vi "prob2.vi"() -> ()   [LabVIEW 2022 SP3]
uses:
  <vilib>/express/express analysis/Spectral/Block/exnSpectralBlock spectral measurements power poly.vi
  <vilib>/express/express analysis/Spectral/Block/exnSpectralBlock spectral measurements power DDT.vi
  <vilib>/express/express analysis/Spectral/XNode/ExpressSpectralMeasurementsBlockNode.xnode
panel:
  in  "stop":bool
  out "Waveform Graph 6":dynamicdata(graph)
  out "Waveform Graph 5":dynamicdata(graph)
  out "Filtered Signal":dynamicdata(graph)
  in  "Cutoff Frequency":dbl(slide) scale=0.0..1000.0
  out "Raw Signal":dynamicdata(graph)
  out "Channel 2":dynamicdata(graph)
  in  "Amplitude":dbl(slide) scale=0.0..10.0
  in  "Frequency":dbl(knob) scale=0.0..1000.0
  out "Channel 1":dynamicdata(graph)
  in  "Amplitude":dbl(slide) scale=0.0..10.0
  in  "Frequency":dbl(knob) scale=0.0..1000.0
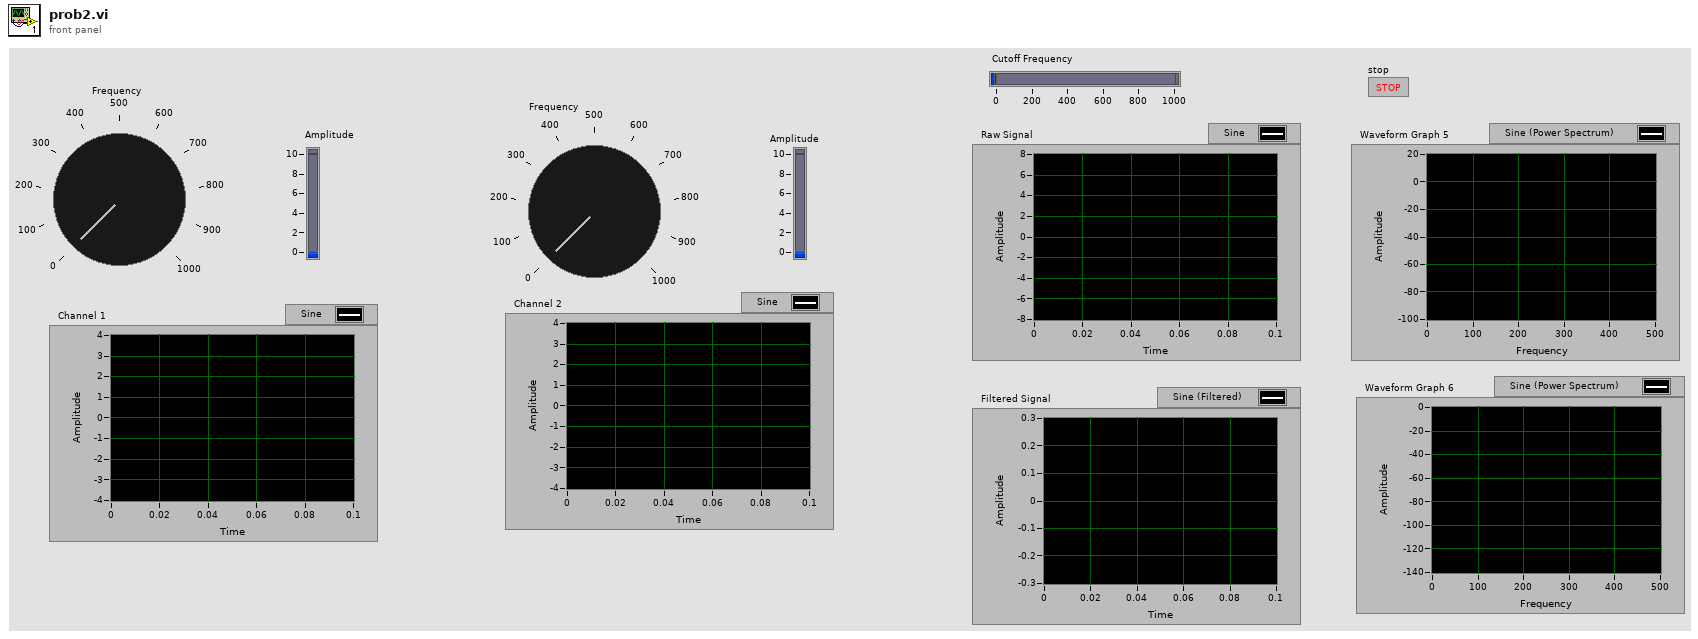
[diagram p1: front panel]
types:
  T1 = cluster{"averaging mode":u16, "weighting mode":u16, "number of averages":u32}
  T2 = cluster{"dB On (F)":bool, "unwrap phase (F)":bool, "convert to degree (F)":bool}
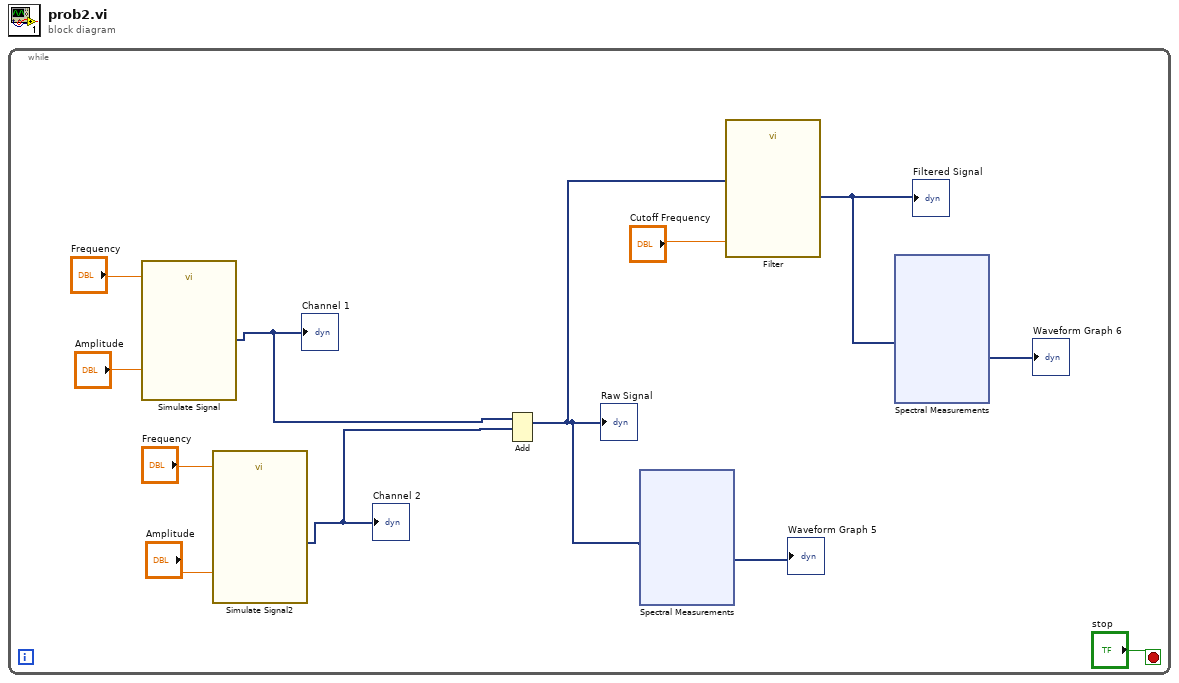
[diagram p0: block diagram]
diagram:
  n1 = while {
    stop <- "stop" stop-if-true
    n2 = call "Simulate Signal"("Frequency"="Frequency", "Amplitude"="Amplitude") -> ("Sine"=w8:dynamicdata)  [unwired: 12 in, 1 out]
    "Channel 1" <- w8
    n3 = call "Simulate Signal2"("Frequency"="Frequency", "Amplitude"="Amplitude") -> ("Sine"=w7:dynamicdata)  [unwired: 12 in, 1 out]
    "Channel 2" <- w7
    n4 = Add(1:w7, 2:w8) -> (0:w5:dynamicdata)  [unwired: 1 in, 1 out]
    "Raw Signal" <- w5
    n5 = xnode "Spectral Measurements"("Signals"=w5) -> ("Power Spectrum"=→"Waveform Graph 5":dynamicdata)  [unwired: 1 in, 1 out]
    n6 = call "Filter"("Lower Cut-Off"="Cutoff Frequency", "Signal"=w5) -> ("Filtered Signal"=w3:dynamicdata)  [unwired: 8 in, 1 out]
    "Filtered Signal" <- w3
    n7 = xnode "Spectral Measurements"("Signals"=w3) -> ("Power Spectrum"=→"Waveform Graph 6":dynamicdata)  [unwired: 1 in, 1 out]
  }
